vi "rad_Apply Network Settings (DHCP).vi"(6 "Timeout in ms (4s)":u32=4000, 8 "error in (no error)":errorcluster, 10 "Requested settings":T1={"Hostname"="", "Serial number"="", "Product name"="", "Product code"=0, "System status"="", "Credential type"=enum."None/Unlocked", "User added?"=FALSE, "Primary NIC"={"MAC address"="", "IP Address Request Mode"=2, "IP address"="", "Subnet mask"="", "Gateway"="", "DNS server"=""}} {"Primary NIC"."IP Address Request Mode" items=["Static"=1, "DHCP/Link-Local"=2, "Link-Local Only"=4, "DHCP Only"=8]}, 11 "Existing settings":T1={"Hostname"="", "Serial number"="", "Product name"="", "Product code"=0, "System status"="", "Credential type"=enum."None/Unlocked", "User added?"=FALSE, "Primary NIC"={"MAC address"="", "IP Address Request Mode"=2, "IP address"="", "Subnet mask"="", "Gateway"="", "DNS server"=""}} {"Primary NIC"."IP Address Request Mode" items=["Static"=1, "DHCP/Link-Local"=2, "Link-Local Only"=4, "DHCP Only"=8]}) -> (0 "error out":errorcluster, 3 "Target settings out":T1={"Hostname"="", "Serial number"="", "Product name"="", "Product code"=0, "System status"="", "Credential type"=enum."None/Unlocked", "User added?"=FALSE, "Primary NIC"={"MAC address"="", "IP Address Request Mode"=2, "IP address"="", "Subnet mask"="", "Gateway"="", "DNS server"=""}} {"Primary NIC"."IP Address Request Mode" items=["Static"=1, "DHCP/Link-Local"=2, "Link-Local Only"=4, "DHCP Only"=8]})   [LabVIEW 2013]
uses:
  TypeDefs/rad_Target Information.ctl
  TypeDefs/rad_Target Network Settings.ctl
  <vilib>/nisyscfg/Save Changes (System).vi
  <vilib>/nisyscfg/Close (System).vi
  <vilib>/nisyscfg/nisyscfg.lvlib
  <resource>/objmgr/nisysapi.rc
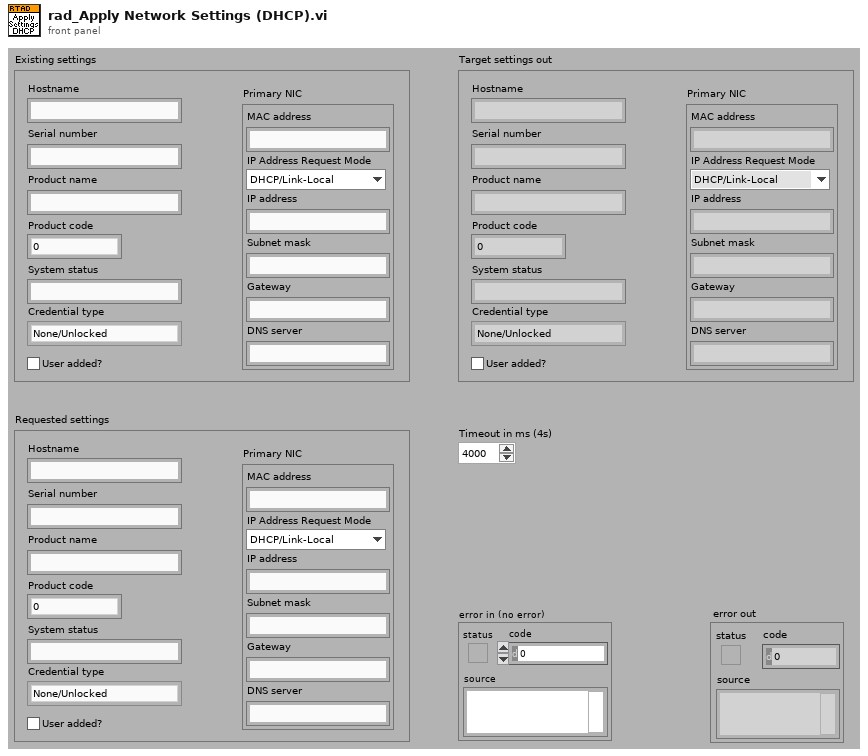
[diagram p1: front panel]
types:
  T1 = typedef "rad_Target Information.ctl" = cluster{"Hostname":string, "Serial number":string, "Product name":string, "Product code":i32, "System status":string, "Credential type":enum16{"None/Unlocked", "FTP Password", "NIAuth Credentials"}, "User added?":bool, "Primary NIC":T2}
  T2 = typedef "rad_Target Network Settings.ctl" = cluster{"MAC address":string, "IP Address Request Mode":i32, "IP address":string, "Subnet mask":string, "Gateway":string, "DNS server":string}
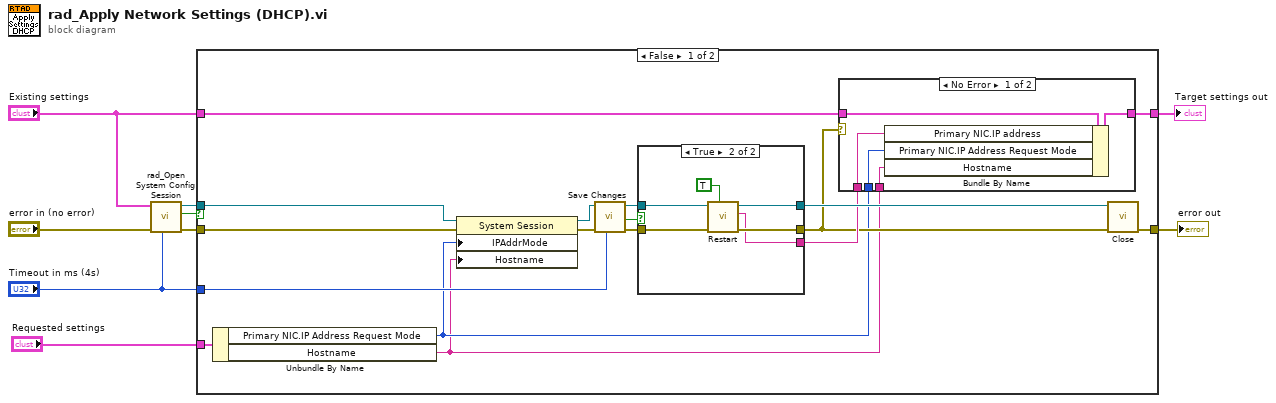
[diagram p0: block diagram]
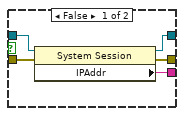
[diagram p3: hidden frame]
diagram:
  n1 = call "rad_Open System Config Session.vi"("Timeout ms (4000)"="Timeout in ms (4s)", "error in (no error)"="error in (no error)", "Target settings"="Existing settings") -> ("error out"=w6:errorcluster, "Cancelled"=w4:bool, "Session out"=w7:refnum<k21>)  [unwired: 5 in, 1 out]
  n2 = case shown="False" w4 {
    tunnel: w7 -> [w26 _]
    tunnel: w6 -> [w25 w45]
    tunnel: [w24 w45] -> w8
    tunnel: "Timeout in ms (4s)" -> [w18 _]
    tunnel: "Existing settings" -> [w17 w44]
    tunnel: [w16 w44] -> w3
    tunnel: "Requested settings" -> [w12 _]
    frame False {
      n3 = Unbundle By Name(w12) -> ("Primary NIC.IP Address Request Mode"=w11:i32, "Hostname"=w10:string)
      n4 = property class="System Session"(reference=w26, error in=w25, "IPAddrMode"=w11, "Hostname"=w10) -> (reference out=w23:refnum<k21>, error out=w22:errorcluster)
      n5 = call-poly <vilib>:"Save Changes.vi"("Remote Timeout (300,000 ms)"=w18, "error in (no error)"=w22, "Session in"=w23) -> ("error out"=w20:errorcluster, "Changes Require Restart"=w21:bool, "Session out"=w19:refnum<k21>)  [unwired: 5 in, 1 out]
      n6 = case shown="True" w21 {
        tunnel: w20 -> [w37 w43]
        tunnel: [w36 w42] -> w13
        tunnel: w19 -> [w35 w41]
        tunnel: [w34 w40] -> w15
        tunnel: [w33 w38] -> w14
        frame False {
          n7 = property class="System Session"(reference=w35, error in=w37) -> (reference out=w34:refnum<k21>, error out=w36:errorcluster, "IPAddr"=w33:string)
        }
        frame True {
          n8 = call <vilib>:"Restart.vi"("Wait Until Complete (T)"=TRUE ("wait until complete (T)"), "error in (no error)"=w43, "Session in"=w41) -> ("error out"=w42:errorcluster, "New IP Address"=w38:string, "Session out"=w40:refnum<k21>)  [unwired: 6 in]
        }
      }
      n9 = case shown="No Error" w13 {
        tunnel: w17 -> [w31 w32]
        tunnel: [w30 w32] -> w16
        tunnel: w10 -> [w29 _]
        tunnel: w11 -> [w28 _]
        tunnel: w14 -> [w27 _]
        frame No Error {
          n10 = Bundle By Name(cluster=w31, "Primary NIC.IP address"=w27, "Primary NIC.IP Address Request Mode"=w28, "Hostname"=w29) -> (w30:T1)
        }
        frame Error {
        }
      }
      n11 = call-poly <vilib>:"Close.vi"("error in (no error)"=w13, "Session in"=w15) -> ("error out"=w24:errorcluster)  [unwired: 9 in]
    }
    frame True {
    }
  }
  "error out" <- w8
  "Target settings out" <- w3
